vi "FarFiledCamConnectCheck.vi"() -> (0 "error out":errorcluster, 1 "通信正常":bool)   [LabVIEW 2018]
panel:
  out "错误报告":string
  out "ReturnValue":u32
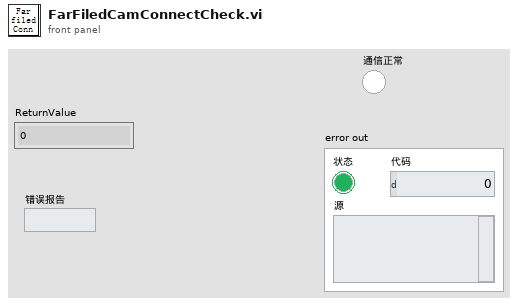
[diagram p1: front panel]
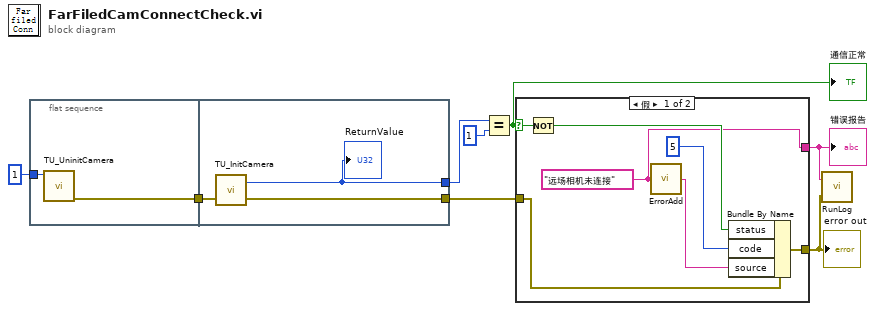
[diagram p0: block diagram]
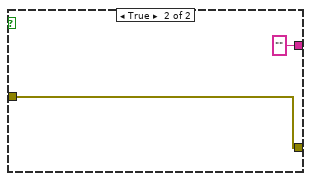
[diagram p2: hidden frame]
diagram:
  n1 = flat-sequence {
    tunnel: u32 1 ("nCamCount") -> [w10]
    tunnel: [w9] -> w7
    tunnel: w7 -> [w13]
    tunnel: [w12] -> w6
    tunnel: [w11] -> w4
    frame #0 {
      n2 = call "TU_UninitCamera.vi"("nCamCount"=w10) -> ("error out"=w9:errorcluster)  [unwired: 8 in, 1 out]
    }
    frame #1 {
      n3 = call "TU_InitCamera.vi"("error in (no error)"=w13) -> ("error out"=w11:errorcluster, "ReturnValue"=w12:u32)  [unwired: 1 in]
      "ReturnValue" <- w12
    }
  }
  n4 = Equal?(x=w6, y=u32 1) -> (x = y?=w1:bool)
  "通信正常" <- w1
  n5 = case shown="假" w1 {
    selector: w1 -> [w19 _]
    tunnel: w4 -> [w20 w22]
    tunnel: [w15 w22] -> w2
    tunnel: [w14 "" ("source")] -> w3
    frame False {
      w14 = "远场相机未连接" ("source")
      n6 = Not(x=w19) -> (.not. x?=w18:bool)
      n7 = call "ErrorAdd.vi"("source"=w14) -> ("Errorout Souce"=w16:string)
      n8 = Bundle By Name(cluster=w20, "status"=w18, "code"=5, "source"=w16) -> (w15:errorcluster)
    }
    frame True {
    }
  }
  "错误报告" <- w3
  "error out" <- w2
  n9 = call "RunLog.vi"("error in"=w2, "Message"=w3) -> ()  [unwired: 1 in, 1 out]
